vi "Configure Data Format.vi"(8 "error in (no error)":errorcluster, 9 "Byte Order (0: Normal)":i32(ring) items=["Normal", "Swapped"], 10 "Data Format (0: Ascii)":i32(ring) items=["Ascii", "Real32", "Real64"], 11 "VISA resource name":refnum<visa-resource-name>) -> (0 "error out":errorcluster, 3 "VISA resource name out":refnum<visa-resource-name>)   [LabVIEW 2018, in "Keysight PNA Series.lvlib"]
doc: "Configures the way that data will be transferred when moving large amounts of data."
uses:
  Keysight PNA Series.lvlib
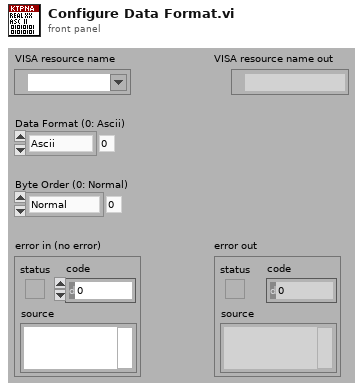
[diagram p1: front panel]
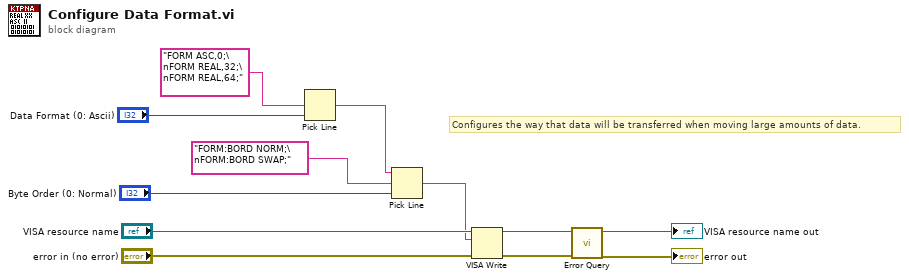
[diagram p0: block diagram]
diagram:
  # "Configures the way that data will be transferred when moving large amounts of data."
  n1 = Pick Line(multi-line string="FORM ASC,0;\nFORM REAL,32;\nFORM REAL,64;", line index="Data Format (0: Ascii)") -> (output string=w2:string)  [unwired: 1 in]
  n2 = Pick Line(string ("")=w2, multi-line string="FORM:BORD NORM;\nFORM:BORD SWAP;", line index="Byte Order (0: Normal)") -> (output string=w1:string)
  n3 = VISA Write(VISA resource name="VISA resource name", write buffer=w1, error in (no error)="error in (no error)") -> (VISA resource name out=w6:refnum<visa-resource-name>, error out=w5:errorcluster)  [unwired: 1 out]
  n4 = call "Error Query.vi"("error in (no error)"=w5, "VISA resource name"=w6) -> ("error out"=→"error out":errorcluster, "VISA resource name out"=→"VISA resource name out":refnum<visa-resource-name>)  [unwired: 6 in, 2 out]
